vi "Start Task.vi"(8 "error in (no error)":errorcluster, 11 "DAQ Actor in":refnum<class "DAQ Actor.lvclass">) -> (0 "error out":errorcluster, 3 "DAQ Actor out":refnum<class "DAQ Actor.lvclass">)   [LabVIEW 2012, in "Data Acquisition.lvlib" / "DAQ Actor.lvclass"]
uses:
  DAQ Actor.lvclass
  DAQ Actor.lvclass/DAQ Actor.ctl
  TCP Server/TCP Writer Messages/Add Wfm Header Msg/Add Wfm Header Msg.lvclass/Add Wfm Header Msg.ctl
  <vilib>/ActorFramework/Message Enqueuer/Message Enqueuer.lvclass/Message Enqueuer.ctl
  <vilib>/ActorFramework/Actor/Actor.lvclass/Actor.ctl
  <vilib>/ActorFramework/Message Enqueuer/Enqueue.vi
  <vilib>/ActorFramework/Message Enqueuer/Init from Existing Queue.vi
  <vilib>/ActorFramework/Message Priority Queue/Priority Enqueue.vi
  TCP Server/TCP Writer Messages/Add Wfm Header Msg/Add Wfm Header Msg.lvclass
  <vilib>/ActorFramework/Message Enqueuer/Message Enqueuer.lvclass
  DAQ Actor Messages/Aquire Msg/Aquire Msg.lvclass
  Class DAQ Task/DAQ Task.lvclass
  <vilib>/ActorFramework/Actor/Actor.lvclass
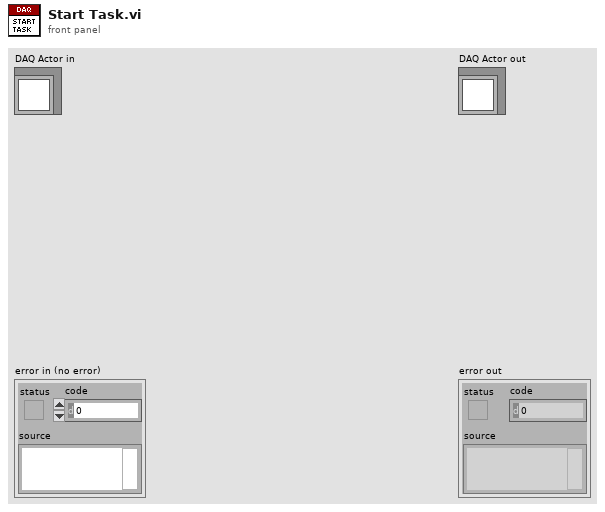
[diagram p1: front panel]
types:
  T1 = typedef "TE_Designator.ctl" = enum16{"High Speed", "Low Speed"}
  T2 = typedef "Waveform Header.ctl" = cluster{"dt":dbl, "attributes (str)":string[][]}
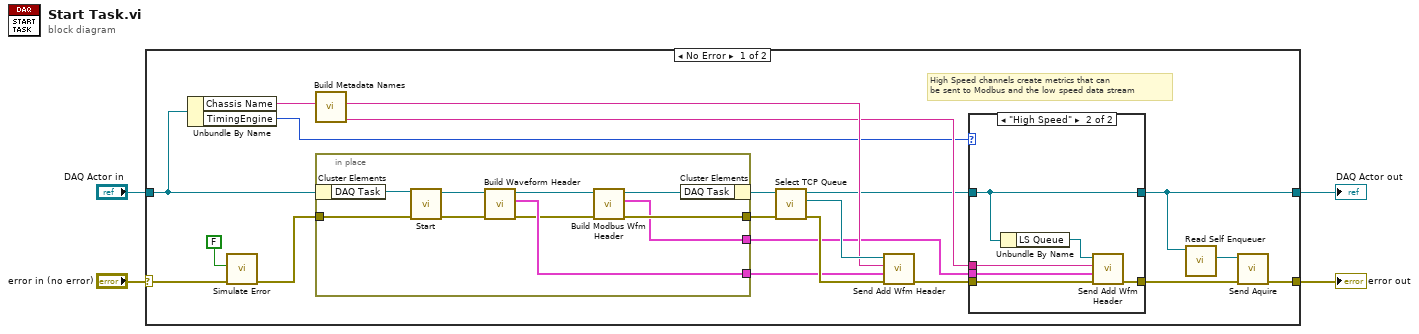
[diagram p0: block diagram]
diagram:
  n1 = case shown="No Error" "error in (no error)" {
    selector: "error in (no error)" -> [w21 w44]
    tunnel: [w24 w44] -> w3
    tunnel: [w6 w43] -> w1
    tunnel: "DAQ Actor in" -> [w15 w43]
    frame No Error {
      # "High Speed channels create metrics that can \nbe sent to Modbus and the low speed data stream"
      n2 = Unbundle By Name(w15) -> ("Chassis Name"=w14:string, "TimingEngine"=w5:T1)
      n3 = call "Simulate Error.vi"("error in (no error)"=w21, "Sim Error?"=FALSE) -> ("error out"=w20:errorcluster)  [unwired: 9 in]
      n4 = call "Build Metadata Names.vi"("Chassis Name"=w14) -> ("Modbus Wfm Hdr"=w8:string, "Wfm Hdr"=w13:string)  [unwired: 6 in, 3 out]
      n5 = in-place {
        in-place-border: w20 -> [w41]
        in-place-border: [w34] -> w18
        in-place-border: [w38] -> w12
        in-place-border: [w33] -> w9
        n6 = in-place-cluster #1(w15) -> ("DAQ Task"=w42:refnum<class "DAQ Task.lvclass">)
        n7 = call "Start.vi"("error in (no error)"=w41, "DAQ Task in"=w42) -> ("error out"=w39:errorcluster, "DAQ Task out"=w40:refnum<class "DAQ Task.lvclass">)  [unwired: 8 in]
        n8 = call "Build Waveform Header.vi"("error in (no error)"=w39, "DAQ Task in"=w40) -> ("error out"=w35:errorcluster, "Wfm Header"=w38:T2, "DAQ Task out"=w37:refnum<class "DAQ Task.lvclass">)  [unwired: 7 in]
        n9 = call "Build Modbus Wfm Header.vi"("error in (no error)"=w35, "DAQ Task in"=w37) -> ("error out"=w34:errorcluster, "Wfm Header"=w33:T2, "DAQ Task out"=w36:refnum<class "DAQ Task.lvclass">)  [unwired: 7 in]
        n10 = in-place-cluster #1("DAQ Task"=w36) -> (w19:refnum<class "DAQ Actor.lvclass">)
      }
      n11 = call "Select TCP Queue.vi"("error in (no error)"=w18, "DAQ Actor in"=w19) -> ("error out"=w16:errorcluster, "TCP Queue"=w17:refnum<class "Message Enqueuer.lvclass">, "DAQ Actor out"=w7:refnum<class "DAQ Actor.lvclass">)  [unwired: 7 in]
      n12 = call "Send Add Wfm Header.vi"("error in (no error)"=w16, "Wfm Header"=w12, "Metadata"=w13, "Message Enqueuer"=w17) -> ("error out"=w10:errorcluster)  [unwired: 6 in, 1 out]
      n13 = case shown="\"High Speed\"" w5 {
        tunnel: [w25 w32] -> w11
        tunnel: w10 -> [w25 w31]
        tunnel: w9 -> [_ w30]
        tunnel: w8 -> [_ w29]
        tunnel: w7 -> [w26 w27]
        tunnel: [w26 w27] -> w6
        frame "Low Speed" {
        }
        frame "High Speed" {
          n14 = Unbundle By Name(w27) -> ("LS Queue"=w28:refnum<class "Message Enqueuer.lvclass">)
          n15 = call "Send Add Wfm Header.vi"("error in (no error)"=w31, "Wfm Header"=w30, "Metadata"=w29, "Message Enqueuer"=w28) -> ("error out"=w32:errorcluster)  [unwired: 6 in, 1 out]
        }
      }
      n16 = call <vilib>:"Read Self Enqueuer.vi"("Actor"=w6) -> ("Self Enqueuer"=w23:refnum<class "Message Enqueuer.lvclass">)  [unwired: 10 in]
      n17 = call "Send Aquire.vi"("error in (no error)"=w11, "Message Enqueuer"=w23) -> ("error out"=w24:errorcluster)  [unwired: 8 in, 1 out]
    }
    frame Error {
    }
  }
  "error out" <- w3
  "DAQ Actor out" <- w1
